vi "PH_Beckhoff-16BB.constructor.vi"(0 "name":string, 2 "data in":string, 5 "error in(no error)":errorcluster) -> (14 "i ref out":refnum<vi>, 16 "data out":string, 19 "error out":errorcluster)   [LabVIEW 2014, in "PH_Beckhoff-16BB.lvlib"]
doc: "This is the constructor of a class.\n\nLicense Agreement for this software:\n\nCopyright (C)\nGesellschaft für Schwerionenforschung, GSI\nPlanckstr. 1\n64291 Darmstadt\nGermany\n\nContact: D.Beck@gsi.de \n\nThis program is free software; you can redistribute it and/or modify it under the terms of the \nGNU General Public License as published by the Free Software Foundation; either version 2 of \nthe license, or (at your option) any later version.\n\nThis program is distributed in the hope that it will be useful, but WITHOUT ANY WARRANTY; \nwithout even the implied warranty of MERCHANTABILITY or FITNESS FOR A PARTICULAR PURPOSE. See the GNU General License for more details (http://www.gnu.org).\n\nGesellschaft für Schwerionenforschung, GSI\nPlanckstr. 1, 64291 Darmstadt, Germany\nFor all questions and ideas contact: M.Richter@gsi.de, H.Brand@gsi.de or D.Beck@gsi.de.\nLast update: 16-JUN-2004"
uses:
  PH_Beckhoff-16BB.lvlib
  PH_Basics/PH_PSDBWriter/PH_PSDBWriter.Thread Commands.ctl
  CS_Core/CSSystem/CSSystemLib/CSSystemLib.lvlib
  PH_Beckhoff/PH_Beckhoff.lvlib
  PH_Basics/PH_PSDBWriter/PH_PSDBWriter.lvlib
  PH_Basics/PH_Class/PH_Class.lvlib
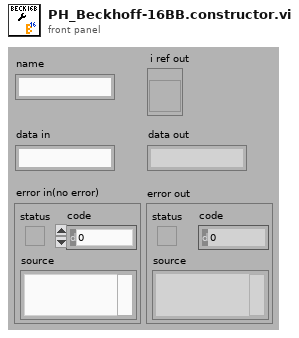
[diagram p1: front panel]
types:
  T1 = enum16{"SetAttribute", "GetAttribute", "CreateAttribute", "DestroyAttribute", "DestroyAllAtributes"}
  T2 = typedef "PH_Beckhoff.lvlib/PH_Beckhoff.constructor Data in.ctl" = cluster{"Default Values":T3, "Description":string, "Hardware configured?":bool, "Activate Change Manager?":bool, "Difference to handle an analog input as change":u32}
  T3 = typedef "PH_Beckhoff.lvlib/PH_Beckhoff.Values.ctl" = cluster{"Sonderklemmen Inputs":T4, "Analog Inputs":T5, "Analog Outputs":T7, "Digital Inputs":T8, "Digital Outputs":T9}
  T4 = typedef "PH_Beckhoff.lvlib/PH_Beckhoff.Sonderklemmen Inputs.ctl" = cluster{"Total Length":u32, "Name":string, "Value":u64, "Quality":bool, "Service ID":i32, "Offset":u32, "Length":u32}[]
  T5 = typedef "PH_Beckhoff.lvlib/PH_Beckhoff.Analog Inputs.ctl" = cluster{"Name":string, "Value":u32, "Quality":bool, "Service ID":i32, "Sca Type":T6}[]
  T6 = typedef "PH_Beckhoff.lvlib/PH_Beckhoff.Scaling Type.ctl" = enum16{"none", "0 ... 15 Bit -> 0 ... 5", "0 ... 15 Bit -> 0 ... 10", "0 ... 15 Bit -> 0 ... 25", "0 ... 15 Bit -> 4 ... 20", "0 ... 15 Bit -> 0 ... 1", "0 ... 15 Bit -> 0 ... 20000", "0 ... 15 Bit -> 0 ... 24000"}
  T7 = typedef "PH_Beckhoff.lvlib/PH_Beckhoff.Analog Outputs.ctl" = cluster{"Name":string, "Value":u32, "Quality":bool, "Wanted Value":u32, "Service ID":i32, "Sca Type":T6}[]
  T8 = typedef "PH_Beckhoff.lvlib/PH_Beckhoff.Digital Inputs.ctl" = cluster{"Name":string, "Value":bool, "Quality":bool, "Service ID":i32, "inverted?":bool}[]
  T9 = typedef "PH_Beckhoff.lvlib/PH_Beckhoff.Digital Outputs.ctl" = cluster{"Name":string, "Value":bool, "Quality":bool, "Wanted Value":bool, "Service ID":i32, "inverted?":bool}[]
  T10 = typedef "PH_Beckhoff-16BB.lvlib/PH_Beckhoff-16BB.i attribute.ctl" = cluster{"PA Chiller":cluster{"PSDB":cluster{"Status Service ID":i32, "Instance ID":i32, "Data Status":T11, "Ref Status":refnum<vi>, "Error Code":i32}, "Status":cluster{"GUI Ref":refnum<vi>, "Status Service ID":i32, "Status":T12}, "DIs":cluster{"Flow Control":cluster{"GUI Ref":refnum<vi>, "# in Data":i32}, "High-Temp":cluster{"GUI Ref":refnum<vi>, "# in Data":i32}, "Conductivity":cluster{"GUI Ref":refnum<vi>, "# in Data":i32}, "Niveau":cluster{"GUI Ref":refnum<vi>, "# in Data":i32}}, "PSDB Thread":cluster{"Ref":refnum<vi>, "Q-Ref":refnum<queue>}}, "PSDB":cluster{"Shot #":i32, "Subsystem":T13}, "Racktype":string, "PSDB Credentials":T14}
  T11 = typedef "PH_PSDBWriter.lvlib/PH_PSDBWriter.Data Status.ctl" = i16
  T12 = typedef "PH_StatusHandler.lvlib/PH_StatusHandler.Status.ctl" = i16
  T13 = typedef "PH_PSDBWriter.lvlib/PH_PSDBWriter.PHELIX-Subsystems.ctl" = i32
  T14 = typedef "PH_Common.lvlib/PH_Connection.PSDB Credentials.ctl" = cluster{"PW":string, "ID":string, "DS":string}
  T15 = typedef "PH_PSDBWriter.lvlib/PH_PSDBWriter.Thread Commands.ctl" = u16
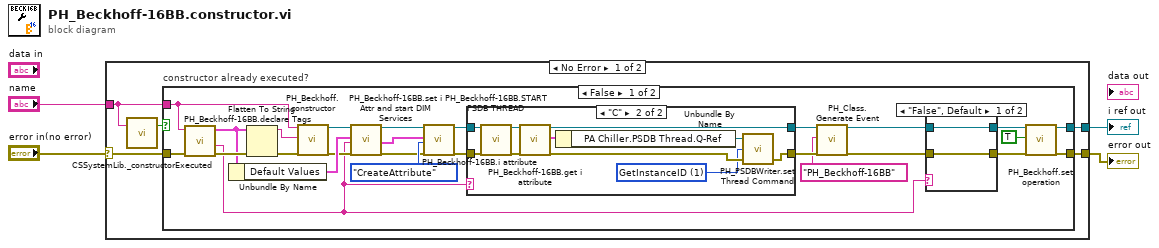
[diagram p0: block diagram]
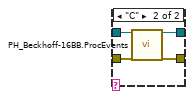
[diagram p2: hidden frame]
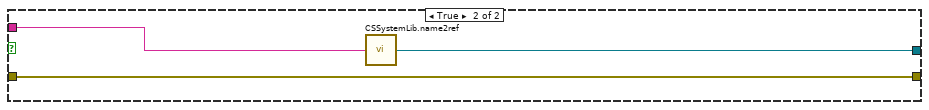
[diagram p4: hidden frame]
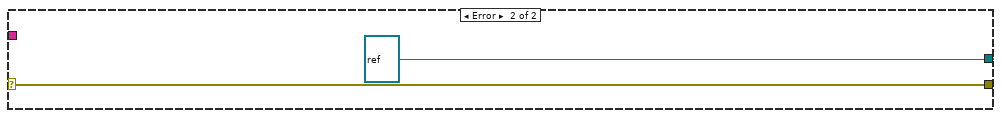
[diagram p5: hidden frame]
diagram:
  n1 = case shown="No Error" "error in(no error)" {
    selector: "error in(no error)" -> [w9 w58]
    tunnel: "name" -> [w8 _]
    tunnel: [w6 refnum<vi> refnum ("obj refnum")] -> w3
    tunnel: [w5 w58] -> w2
    frame No Error {
      n2 = call "CSSystemLib._constructorExecuted.vi"("name"=w8) -> ("constructor executed?"=w7:bool)  [unwired: 18 in]
      n3 = case "constructor already executed?" shown="False" w7 {
        tunnel: [w32 w55] -> w6
        tunnel: [w31 w54] -> w5
        tunnel: w9 -> [w28 w54]
        tunnel: w8 -> [w29 w56]
        frame False {
          n4 = call "PH_Beckhoff-16BB.declare Tags.vi"("error in (no error)"=w28, "Instance Name"=w29) -> ("error out"=w30:errorcluster, "Racktype"=w10:string, "Data in cluster"=w18:T2)  [unwired: 3 in]
          n5 = Unbundle By Name(w18) -> ("Default Values"=w26:T3)
          n6 = Flatten To String(anything=w18, error in (no error)=w30) -> (data string=w35:string, error out=w34:errorcluster)  [unwired: 2 in, 1 out]
          n7 = call "PH_Beckhoff.constructor.vi"("name"=w29, "data in"=w35, "error in(no error)"=w34) -> ("i ref out"=w21:refnum<vi>, "error out"=w22:errorcluster)  [unwired: 14 in, 1 out]
          n8 = call "PH_Beckhoff-16BB.set i Attr and start DIM Services.vi"("i ref in"=w21, "Values"=w26, "Racktype"=w10, "error in"=w22) -> ("i ref out"=w25:refnum<vi>, "i Attr"=w23:T10, "error out"=w24:errorcluster)  [unwired: 13 in]
          n9 = call "PH_Beckhoff-16BB.i attribute.vi"("VI Refnum"=w25, "CLASS.i attribute"=w23, "Action"=T1."CreateAttribute", "error in (no error)"=w24) -> ("VI Refnum out"=w20:refnum<vi>, "error out"=w19:errorcluster)  [unwired: 13 in, 1 out]
          n10 = case shown="\"C\"" w10 {
            tunnel: w19 -> [w42 w46]
            tunnel: [w42 w44] -> w16
            tunnel: w20 -> [w43 w47]
            tunnel: [w43 w45] -> w15
            frame Default {
            }
            frame "C" {
              w50 = T15 1 items=["None", "GetInstanceID", "WriteToPSDB"] ("PSDB Thread Command")
              n11 = call "PH_Beckhoff-16BB.START PSDB THREAD.vi"("VI in"=w47, "error in (no error)"=w46) -> ("VI out"=w49:refnum<vi>, "error out"=w48:errorcluster)  [unwired: 16 in]
              n12 = call "PH_Beckhoff-16BB.get i attribute.vi"("i ref in"=w49, "error in (no error)"=w48) -> ("i ref out"=w45:refnum<vi>, "i attribute"=w52:T10, "error out"=w53:errorcluster)  [unwired: 15 in]
              n13 = Unbundle By Name(w52) -> ("PA Chiller.PSDB Thread.Q-Ref"=w51:refnum<queue>)
              n14 = call "PH_PSDBWriter.set Thread Command.vi"("error in (no error)"=w53, "PSDB Thread Command"=w50, "Queue in"=w51) -> ("error out"=w44:errorcluster)  [unwired: 2 in]
            }
          }
          n15 = call "PH_Class.Generate Event.vi"("i ref in"=w15, "Class"="PH_Beckhoff-16BB", "error in (no error)"=w16) -> ("i ref out"=w14:refnum<vi>, "error out"=w17:errorcluster)  [unwired: 15 in]
          n16 = case shown="\"False\", Default" w10 {
            tunnel: w17 -> [w36 w41]
            tunnel: w14 -> [w37 w40]
            tunnel: [w37 w39] -> w13
            tunnel: [w36 w38] -> w12
            frame "False", Default {
            }
            frame "C" {
              n17 = call "PH_Beckhoff-16BB.ProcEvents.vi"("i ref in"=w40, "error in"=w41) -> ("i ref out"=w39:refnum<vi>, "error out"=w38:errorcluster)  [unwired: 16 in]
            }
          }
          n18 = call "PH_Beckhoff.set operation.vi"("VI in"=w13, "operation?"=TRUE, "error in (no error)"=w12) -> ("VI out"=w32:refnum<vi>, "error out"=w31:errorcluster)  [unwired: 15 in]
        }
        frame True {
          n19 = call "CSSystemLib.name2ref.vi"("name"=w56) -> ("obj refnum"=w55:refnum<vi>)
        }
      }
    }
    frame Error {
    }
  }
  "i ref out" <- w3
  "error out" <- w2
